vi "Read value (Numeric).vi"(8 "error in (no error)":errorcluster, 9 "default value":dbl, 11 "JSON Numeric in":refnum<class "JSON Value.lvclass">) -> (0 "error out":errorcluster, 1 "defaulted?":bool, 2 "value":dbl)   [LabVIEW 2016, in "JSON Value.lvclass"]
doc: "Returns the value of a JSON Numeric"
uses:
  JSON Value.lvclass
  JSON Value.lvclass/JSON Value.ctl
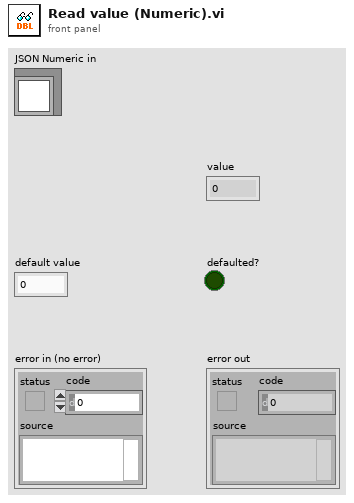
[diagram p1: front panel]
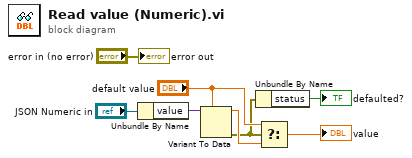
[diagram p0: block diagram]
diagram:
  n1 = Unbundle By Name("JSON Numeric in") -> ("value"=w3:variant)
  n2 = Variant To Data(type="default value", Variant=w3) -> (data=w2:dbl, error out=w1:errorcluster)  [unwired: 1 in]
  n3 = Unbundle By Name(w1) -> ("status"=→"defaulted?":bool)
  n4 = Select(t="default value", s=w1, f=w2) -> (s? t:f=→"value":dbl)
  "error out" <- "error in (no error)"
